vi "uuid.vi"() -> (3 "UUID":string)   [LabVIEW 2014, in "JKI State Machine++.lvlib"]
doc: "Generate <b>Universally Unique Identifier(UUID)</b> according to the standard methods. For example:\n\n - 59703F3AD837\n - 106A470BA5EC\n - 9B781DB313AF\n\n<b>Inputs:</b>\n - N/A\n\n<b>Outputs:</b>\n - <b>UUID</b>: Generated UUID"
uses:
  JKI State Machine++.lvlib
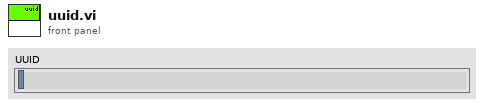
[diagram p1: front panel]
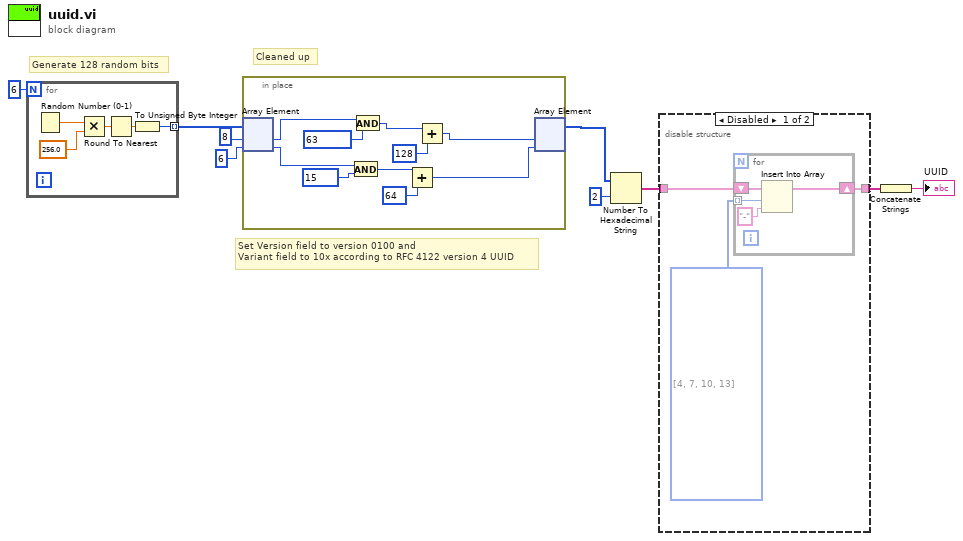
[diagram p0: block diagram]
diagram:
  # "Cleaned up"
  # "Set Version field to version 0100 and \nVariant field to 10x according to RFC 4122 version 4 UUID"
  # "Generate 128 random bits"
  n1 = for {
    N: 6 -> [_]
    tunnel: [w10] -> w8 mode=indexing
    n2 = Random Number (0-1)() -> (number: 0 to 1=w14:dbl)
    n3 = Multiply(x=w14, y=256.0) -> (x*y=w12:dbl)
    n4 = Round To Nearest(number=w12) -> (nearest integer value=w11:dbl)
    n5 = To Unsigned Byte Integer(number=w11) -> (unsigned 8bit integer=w10:u8)
  }
  n6 = in-place {
    n7 = in-place-array #1(w8, 8 ("index"), 6 ("index")) -> (w23:u8, w22:u8)
    n8 = And(x=w22, y=u8 15) -> (x .and. y?=w19:u8)
    n9 = And(x=w23, y=u8 63) -> (x .and. y?=w17:u8)
    n10 = Add(x=w19, y=u8 64) -> (x+y=w15:u8)
    n11 = Add(x=w17, y=u8 128) -> (x+y=w16:u8)
    n12 = in-place-array #1(w16, w15) -> (w4:u8[])  [unwired: 2 out]
  }
  n13 = Number To Hexadecimal String(1:i16 2 ("width (-)"), 2:w4) -> (0:w6:string[])
  n14 = disable-structure shown="Disabled" {
    disable-tunnel: w6 -> [w27 w32]
    disable-tunnel: [w26 w32] -> w5
    frame Disabled {
      n15 = for {
        shift-right: [w30] -> w26
        shift-left: w27 -> [w31]
        tunnel: i32[] [4, 7, 10, 13] ("Array") -> [w28] mode=indexing
        n16 = Insert Into Array(array=w31, index=w28, new element="-" ("new element/subarray")) -> (w30:string[])
      }
    }
    frame Enabled {
    }
  }
  n17 = Concatenate Strings(w5) -> (→"UUID":string)
